vi "PM-A-Acquisition_main_Serial.vi"(8 "error in":errorcluster, 11 "init_cluster":T1) -> (0 "error out":errorcluster)   [LabVIEW 2020]
uses:
  init-close/PM-init-data_cluster.ctl
  init-close/PM-init-user_events.ctl
  init-close/PM-common-heartrate_data.ctl
  init-close/PM-common-peak-detect_settings.ctl
  PM-A-aqn_loop_data.ctl
panel:
  in  "aqn?":bool
  in  "Stop":bool
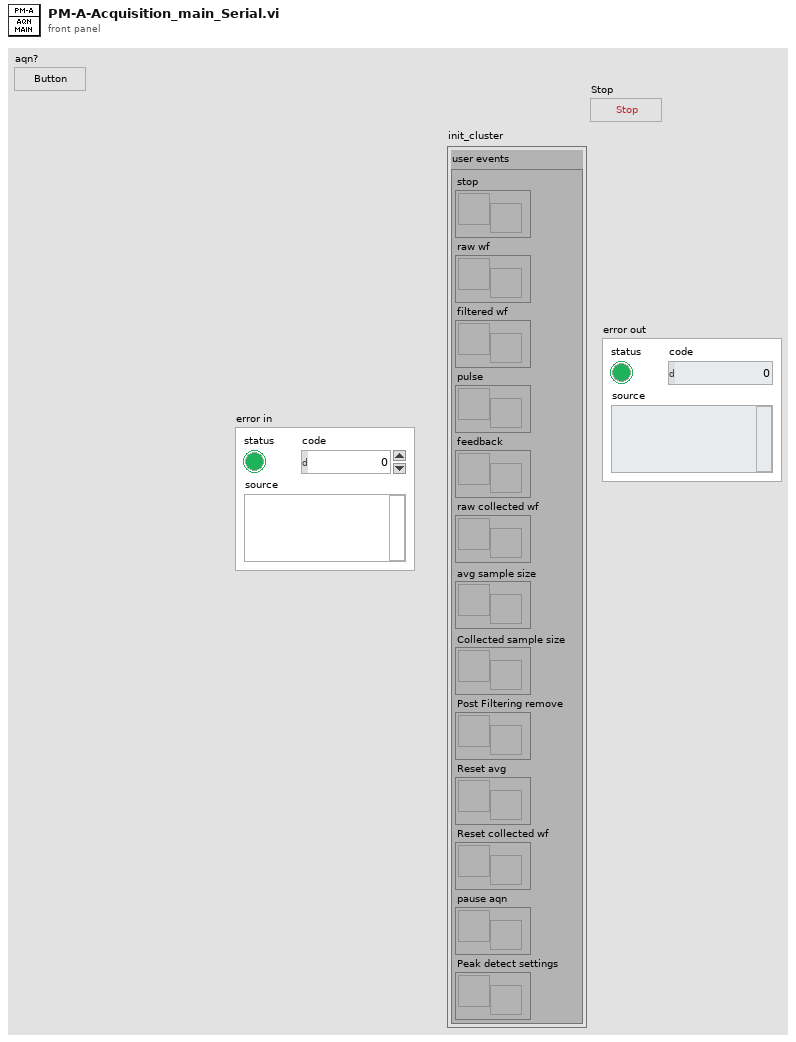
[diagram p1: front panel]
types:
  T1 = typedef "PM-init-data_cluster.ctl" = cluster{"user events":T2}
  T2 = typedef "PM-init-user_events.ctl" = cluster{"stop":refnum<user-event>, "raw wf":refnum<user-event>, "filtered wf":refnum<user-event>, "pulse":refnum<user-event>, "feedback":refnum<user-event>, "raw collected wf":refnum<user-event>, "avg sample size":refnum<user-event>, "Collected sample size":refnum<user-event>, "Post Filtering remove":refnum<user-event>, "Reset avg":refnum<user-event>, "Reset collected wf":refnum<user-event>, "pause aqn":refnum<user-event>, "Peak detect settings":refnum<user-event>}
  T3 = typedef "PM-A-aqn_loop_data.ctl" = cluster{"Stop event":refnum<user-event>, "Raw wf event":refnum<user-event>}
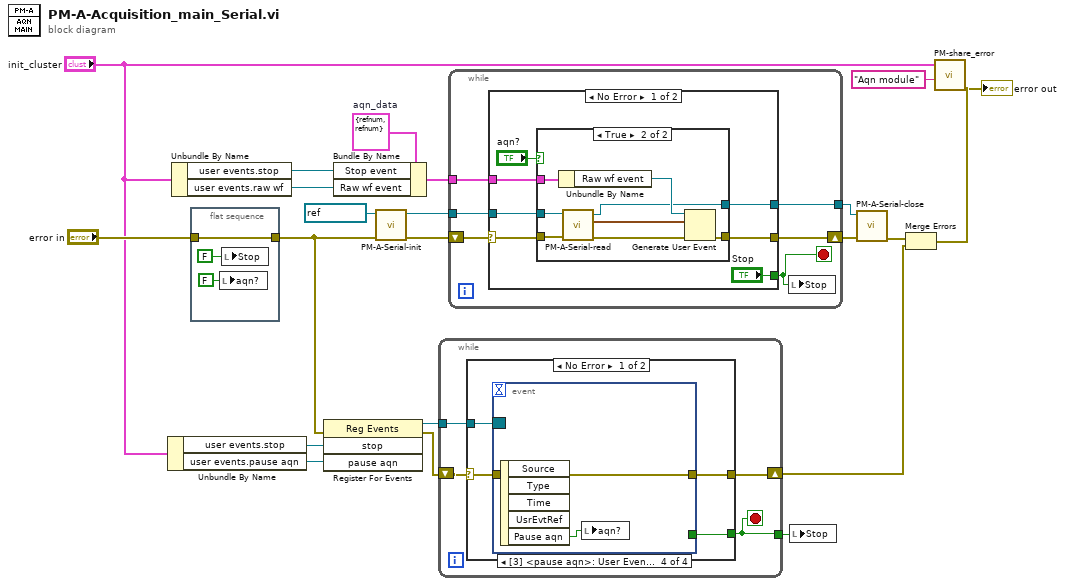
[diagram p0: block diagram]
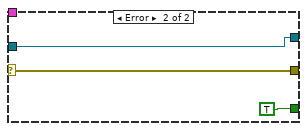
[diagram p3: hidden frame]
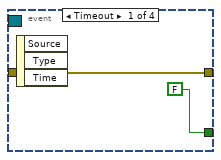
[diagram p4: hidden frame]
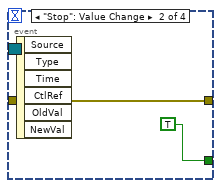
[diagram p5: hidden frame]
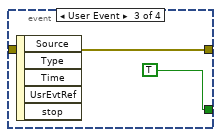
[diagram p6: hidden frame]
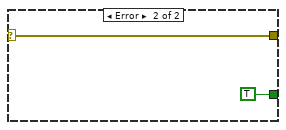
[diagram p7: hidden frame]
diagram:
  w17 = T3 {"Stop event"=refnum, "Raw wf event"=refnum}  # aqn_data
  n1 = Unbundle By Name("init_cluster") -> ("user events.stop"=w19:refnum<user-event>, "user events.pause aqn"=w8:refnum<user-event>)
  n2 = Unbundle By Name("init_cluster") -> ("user events.stop"=w15:refnum<user-event>, "user events.raw wf"=w14:refnum<user-event>)
  n3 = flat-sequence {
    tunnel: "error in" -> [w24]
    tunnel: [w24] -> w7
    frame #0 {
      n4 = local write "aqn?"(FALSE ("aqn?")) -> ()
      n5 = local write "Stop"(FALSE ("Stop")) -> ()
    }
  }
  n6 = register-events(error in=w7, w19, w8) -> (reference out=w18:refnum<event-registration>, error out=w20:errorcluster)  [unwired: 1 in]
  n7 = Bundle By Name(cluster=w17, "Stop event"=w15, "Raw wf event"=w14) -> (w16:T3)
  n8 = call "PM-A-Serial-init.vi"("error in"=w7, "VISA resource name"=refnum<visa-resource-name> "COM5") -> ("error out"=w6:errorcluster, "VISA resource name out"=w4:refnum<visa-resource-name>)  [unwired: 8 in]
  n9 = while {
    tunnel: [w28] -> w22
    shift-right: [w27] -> w21
    shift-left: w20 -> [w29]
    tunnel: w18 -> [w26]
    stop <- w28 stop-if-true
    n10 = case shown="No Error" w29 {
      selector: w29 -> [w31 w42]
      tunnel: [w33 TRUE] -> w28
      tunnel: [w32 w42] -> w27
      tunnel: w26 -> [w30 _]
      frame No Error {
        n11 = event shown="[3] <pause aqn>: User Event" {
          selector: w30 -> [_ _ _ _]
          dyn-events: _ -> [_ _ _ _]
          timeout: _ -> [_ _ _ _]
          tunnel: [FALSE TRUE TRUE _] -> w33
          tunnel: [w34 w37 w39 w41] -> w32
          tunnel: w31 -> [w34 w37 w39 w41]
          event Timeout {
            n12 = event-data() -> ()  [unwired: 1 in, 3 out]
          }
          event "Stop": Value Change {
            n13 = event-data() -> ()  [unwired: 1 in, 6 out]
          }
          event User Event {
            n14 = event-data() -> ()  [unwired: 1 in, 5 out]
          }
          event User Event {
            n15 = event-data() -> ("Pause aqn"=w40:bool)  [unwired: 1 in, 4 out]
            n16 = local write "aqn?"(w40) -> ()
          }
        }
      }
      frame Error {
      }
    }
  }
  n17 = while {
    shift-right: [w48] -> w3
    shift-left: w6 -> [w49]
    tunnel: w16 -> [w46]
    tunnel: w4 -> [w45]
    tunnel: [w44] -> w1
    stop <- w47 stop-if-true
    n18 = case shown="No Error" w49 {
      selector: w49 -> [w55 w69]
      tunnel: ["Stop" TRUE ("Stop")] -> w47
      tunnel: [w54 w69] -> w48
      tunnel: w46 -> [w53 _]
      tunnel: w45 -> [w51 w67]
      tunnel: [w50 w67] -> w44
      frame No Error {
        n19 = case shown="True" "aqn?" {
          tunnel: w55 -> [w58 w62]
          tunnel: [w58 w66] -> w54
          tunnel: w53 -> [_ w65]
          tunnel: w51 -> [w57 w63]
          tunnel: [w57 w59] -> w50
          frame False {
          }
          frame True {
            n20 = Unbundle By Name(w65) -> ("Raw wf event"=w64:refnum<user-event>)
            n21 = call "PM-A-Serial-read.vi"("error in (no error)"=w62, "VISA resource name in"=w63) -> ("error out"=w60:errorcluster, "data"=w61:waveform(dbl), "VISA resource name out"=w59:refnum<visa-resource-name>)  [unwired: 7 in]
            n22 = Generate User Event(user event=w64, event data cluster=w61, error in=w60) -> (error out=w66:errorcluster)  [unwired: 1 in, 1 out]
          }
        }
      }
      frame Error {
      }
    }
    n23 = local write "Stop"(w47) -> ()
  }
  n24 = local write "Stop"(w22) -> ()
  n25 = call "PM-A-Serial-close.vi"("error in (no error)"=w3, "VISA resource name"=w1) -> ("error out"=w2:errorcluster)  [unwired: 9 in]
  n26 = Merge Errors(w2, w21) -> (w12:errorcluster)
  n27 = call "PM-share_error.vi"("error in (no error)"=w12, "module name"="Aqn module", "init_cluster"="init_cluster") -> ("error out"=→"error out":errorcluster)  [unwired: 8 in]
